vi "Test Log Info Message.vi"(8 "error in (no error)":errorcluster, 11 "Test Case In":refnum<class "Logger Test.lvclass">) -> (0 "error out":errorcluster, 3 "Test Case Out":refnum<class "Logger Test.lvclass">)   [LabVIEW 2020, in "Logger Test.lvclass"]
uses:
  Logger Test.lvclass
  Logger Test.lvclass/Logger Test.ctl
  source/Framework Test Suite/Mock Log Handler/Mock Log Handler.lvclass
  source/Framework/Process/Process.lvclass
  source/Framework Test Suite/Mock Process/Mock Process.lvclass
  C:/Git/astemes-triarc-framework/source/Framework/Process/Process.lvclass
  C:/Git/astemes-triarc-framework/source/Framework/Base/Base.lvclass
  C:/Git/astemes-triarc-framework/source/Framework/Configuration File/Configuration File.lvclass
  C:/Git/astemes-triarc-framework/source/Framework/Configuration/Configuration.lvclass
  C:/Git/astemes-triarc-framework/source/Framework/Error Handler Interface/Error Handler Interface.lvclass
  C:/Git/astemes-triarc-framework/source/Framework/Logging/Logging.lvclass
  C:/Git/astemes-triarc-framework/source/Framework Test Suite/Mock Process/Mock Process.lvclass
  C:/Git/astemes-triarc-framework/source/Framework/Async Handler/Async Handler.lvclass
  C:/Git/astemes-triarc-framework/source/Framework/Helper Loop/Helper Loop.lvclass
  source/Framework/Logging/Logging.lvclass
  b13d104d-c40c-48f7-a27a-310fd2f41115.vi
  C:/Git/astemes-triarc-framework/source/Framework Test Suite/Mock Log Handler/Mock Log Handler.lvclass
  b6ab4efb-eff9-46bd-9423-6199dcf06a90.vi
  9b7da4c1-4a3e-432d-b554-2790eb434145.vi
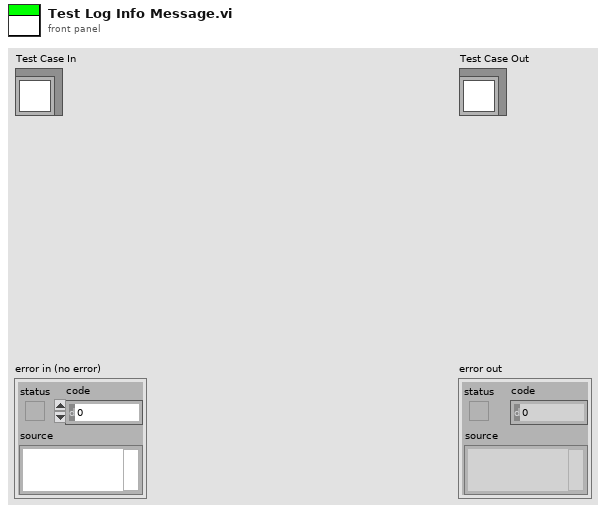
[diagram p1: front panel]
types:
  T1 = typedef "Mock Log Handler.lvclass/Log Entry.ctl" = cluster{"Level":string, "Source":string, "Message":string}
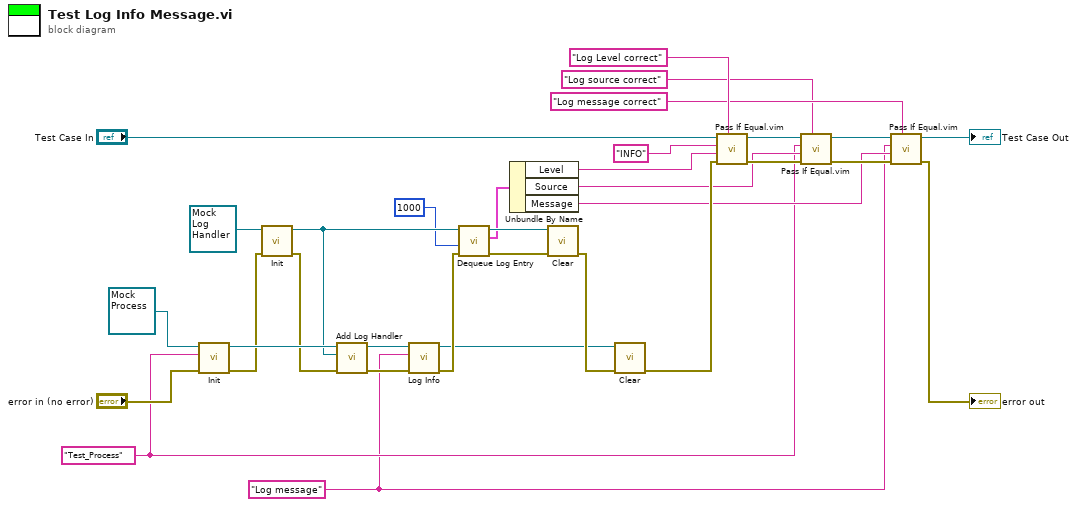
[diagram p0: block diagram]
diagram:
  w2 = "Log message" ("Message")
  w3 = "Test_Process" ("Name")
  n1 = call-dynamic "Init.vi"("error in (no error)"="error in (no error)", "Name"=w3, "Mock Process In"=refnum<class "Mock Process.lvclass"> refnum) -> ("error out"=w25:errorcluster, "Mock Process Out"=w30:refnum<class "Mock Process.lvclass">)  [unwired: 7 in]
  n2 = call-dynamic "Init.vi"("error in (no error)"=w25, "Mock Log Handler In"=refnum<class "Mock Log Handler.lvclass"> refnum ("Mock Log Handler.lvclass")) -> ("error out"=w24:errorcluster, "Mock Log Handler Out"=w21:refnum<class "Mock Log Handler.lvclass">)  [unwired: 8 in]
  n3 = call "Add Log Handler.vi"("error in (no error)"=w24, "Log Handler"=w21, "Process In"=w30) -> ("error out"=w29:errorcluster, "Process Out"=w19:refnum<class "Mock Process.lvclass">)  [unwired: 7 in]
  n4 = call "Log Info.vi"("error in (no error)"=w29, "Message"=w2, "Logging In"=w19) -> ("error out"=w18:errorcluster, "Logging Out"=w1:refnum<class "Mock Process.lvclass">)  [unwired: 7 in]
  n5 = call "Dequeue Log Entry.vi"("error in (no error)"=w18, "timeout in ms (-1)"=1000, "Mock Log Handler in"=w21) -> ("error out"=w22:errorcluster, "Entry"=w16:T1, "Mock Log Handler out"=w23:refnum<class "Mock Log Handler.lvclass">)  [unwired: 5 in, 1 out]
  n6 = Unbundle By Name(w16) -> ("Level"=w15:string, "Source"=w5:string, "Message"=w4:string)
  n7 = call-dynamic "Clear.vi"("error in (no error)"=w22, "Mock Log Handler In"=w23) -> ("error out"=w17:errorcluster)  [unwired: 9 in]
  n8 = call-dynamic "Clear.vi"("error in (no error)"=w17, "Mock Process In"=w1) -> ("error out"=w9:errorcluster)  [unwired: 9 in]
  n9 = call "Pass If Equal.vim"("Description"="Log Level correct", "error in (no error)"=w9, "Actual"=w15, "Expected"="INFO", "LUnit Test Case In"="Test Case In") -> ("error out"=w11:errorcluster, "LUnit Test Case Out"=w32:refnum<class "Logger Test.lvclass">)  [unwired: 5 in]
  n10 = call "Pass If Equal.vim"("Description"="Log source correct", "error in (no error)"=w11, "Actual"=w5, "Expected"=w3, "LUnit Test Case In"=w32) -> ("error out"=w10:errorcluster, "LUnit Test Case Out"=w13:refnum<class "Logger Test.lvclass">)  [unwired: 5 in]
  n11 = call "Pass If Equal.vim"("Description"="Log message correct", "error in (no error)"=w10, "Actual"=w4, "Expected"=w2, "LUnit Test Case In"=w13) -> ("error out"=→"error out":errorcluster, "LUnit Test Case Out"=→"Test Case Out":refnum<class "Logger Test.lvclass">)  [unwired: 5 in]
